vi "calculate channel change_OLD.vi"(0 "set card":i32, 1 "set channel":i32, 2 "current Card":i32, 3 "current Channel":i32, 4 "current card type":string, 5 "set Card Type":string) -> (14 "action":string, 16 "keystrokes":string, 18 "Channels difference":i32)   [LabVIEW 2015]
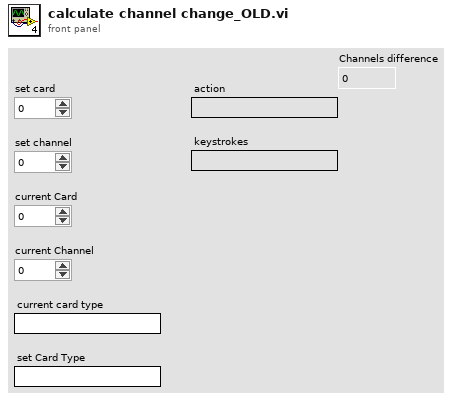
[diagram p1: front panel]
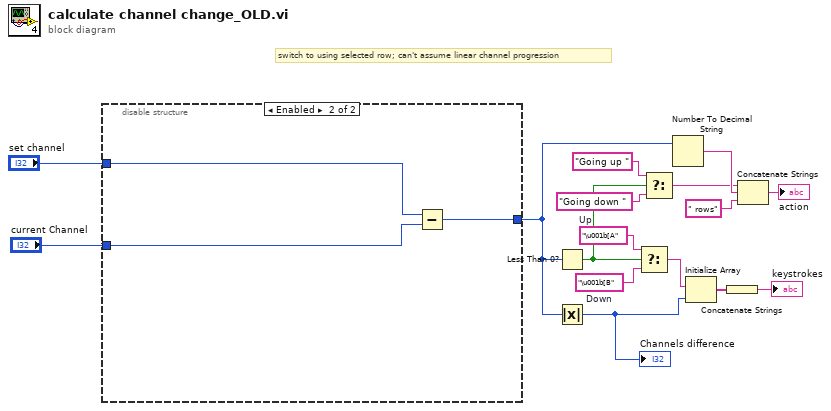
[diagram p0: block diagram]
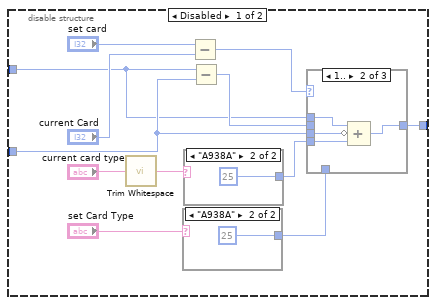
[diagram p2: hidden frame]
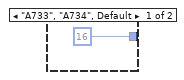
[diagram p3: hidden frame]
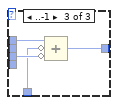
[diagram p5: hidden frame]
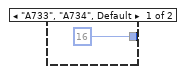
[diagram p6: hidden frame]
diagram:
  w4 = "\u001b[A"  # Up
  w3 = "\u001b[B"  # Down
  # "switch to using selected row; can't assume linear channel progression"
  n1 = disable-structure shown="Enabled" {
    disable-tunnel: [w24 w44] -> w12
    disable-tunnel: "current Channel" -> [w18 w42]
    disable-tunnel: "set channel" -> [w17 w43]
    frame Disabled {
      n2 = call <vilib>:"Trim Whitespace.vi"("string"="current card type") -> ("trimmed string"=w20:string)  [unwired: 1 in]
      n3 = case shown="\"A938A\"" "set Card Type" {
        tunnel: [16 ("set card") 25 ("set card")] -> w23
        frame "A733", "A734", Default {
        }
        frame "A938A" {
        }
      }
      n4 = case shown="\"A938A\"" w20 {
        tunnel: [16 ("set card") 25 ("set card")] -> w22
        frame "A733", "A734", Default {
        }
        frame "A938A" {
        }
      }
      n5 = Subtract(x="set card", y="current Card") -> (x-y=w27:i32)
      n6 = Subtract(x=w17, y=w18) -> (x-y=w28:i32)
      n7 = case shown="1.." w27 {
        tunnel: w18 -> [_ w32 w39]
        tunnel: w22 -> [_ w33 _]
        tunnel: [w31 w35 w38] -> w24
        tunnel: w28 -> [w31 _ _]
        tunnel: w17 -> [_ w34 w36]
        tunnel: w23 -> [_ _ w37]
        frame 0 {
        }
        frame 1.. {
          n8 = Compound Arithmetic op=ADD(w34, invert w32, w33) -> (w35:i32)
        }
        frame ..-1 {
          n9 = Compound Arithmetic op=ADD(w36, invert w37, invert w39) -> (w38:i32)
        }
      }
    }
    frame Enabled {
      n10 = Subtract(x=w43, y=w42) -> (x-y=w44:i32)
    }
  }
  n11 = Less Than 0?(x=w12) -> (x < 0?=w10:bool)
  n12 = Absolute Value(x=w12) -> (abs(x)=w8:i32)
  "Channels difference" <- w8
  n13 = Select(t=w4, s=w10, f=w3) -> (s? t:f=w5:string)
  n14 = Select(t="Going up " ("Up"), s=w10, f="Going down " ("Down")) -> (s? t:f=w13:string)
  n15 = Number To Decimal String(number=w12) -> (decimal integer string=w14:string)  [unwired: 1 in]
  n16 = Initialize Array(w5, w8) -> (w6:string[])
  n17 = Concatenate Strings(w6) -> (→"keystrokes":string)
  n18 = Concatenate Strings(w13, w14, " rows" ("Down")) -> (→"action":string)
